vi "Close.vi"(8 "error in":errorcluster, 11 "TDMS Sink in":refnum<class "TDMS Sink.lvclass">) -> (0 "error out":errorcluster, 3 "TDMS Sink out":refnum<class "TDMS Sink.lvclass">)   [LabVIEW 2024, in "TDMS Sink.lvclass"]
uses:
  TDMS Sink.lvclass
  TDMS Sink.lvclass/TDMS Sink.ctl
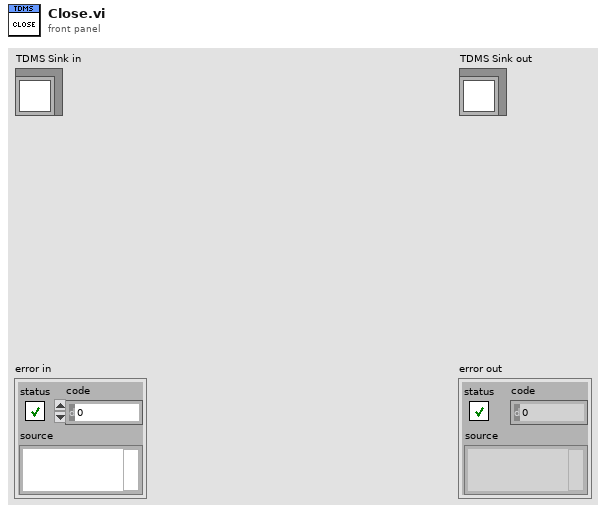
[diagram p1: front panel]
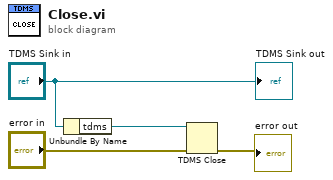
[diagram p0: block diagram]
diagram:
  n1 = Unbundle By Name("TDMS Sink in") -> ("tdms"=w1:refnum<k34>)
  n2 = TDMS Close(8:"error in", 11:w1) -> (0:→"error out":errorcluster)  [unwired: 1 out]
  "TDMS Sink out" <- "TDMS Sink in"
